vi "GetPages.vi"(8 "error in":errorcluster, 11 "PageSelector in":refnum<class "PageSelector.lvclass">) -> (0 "error out":errorcluster, 3 "PageSelector out":refnum<class "PageSelector.lvclass">)   [LabVIEW 2014, in "Raspberry Pi Compatible Compiler for LabVIEW.lvlib" / "PageSelector.lvclass"]
uses:
  PageSelector.lvclass
  PageSelector.lvclass/PageSelector.ctl
  Page/Page.lvclass
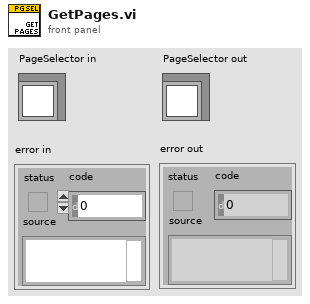
[diagram p1: front panel]
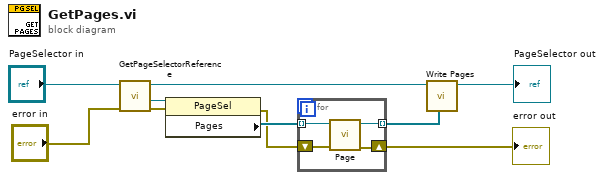
[diagram p0: block diagram]
diagram:
  n1 = call "GetPageSelectorReference.vi"("error in"="error in", "PageSelector in"="PageSelector in") -> ("error out"=w7:errorcluster, "page selector reference"=w8:refnum<vi>, "PageSelector out"=w4:refnum<class "PageSelector.lvclass">)  [unwired: 7 in]
  n2 = property class="PageSel"(reference=w8, error in=w7) -> (error out=w5:errorcluster, "Pages"=w6:refnum<vi>[])  [unwired: 1 out]
  n3 = for {
    tunnel: w6 -> [w13] mode=indexing
    shift-right: [w11] -> w2
    shift-left: w5 -> [w14]
    tunnel: [w12] -> w3 mode=indexing
    n4 = call "Page.vi"("error in"=w14, "Gen Refnum"=w13) -> ("error out"=w11:errorcluster, "Page out"=w12:refnum<class "Page.lvclass">)  [unwired: 8 in]
  }
  "error out" <- w2
  n5 = call "Write Pages.vi"("Pages"=w3, "PageSelector in"=w4) -> ("PageSelector out"=→"PageSelector out":refnum<class "PageSelector.lvclass">)  [unwired: 7 in]
